vi "UI-SelfCheck.vi"() -> ()   [LabVIEW 2014]
panel:
  in  "error in (no error)":errorcluster caption="错误输入（无错误）"
  out "error out":errorcluster caption="错误输出"
  out "数据采集系统":string
  out "拖动系统":string
  out "齿轮系统":string
  out "液压系统":string
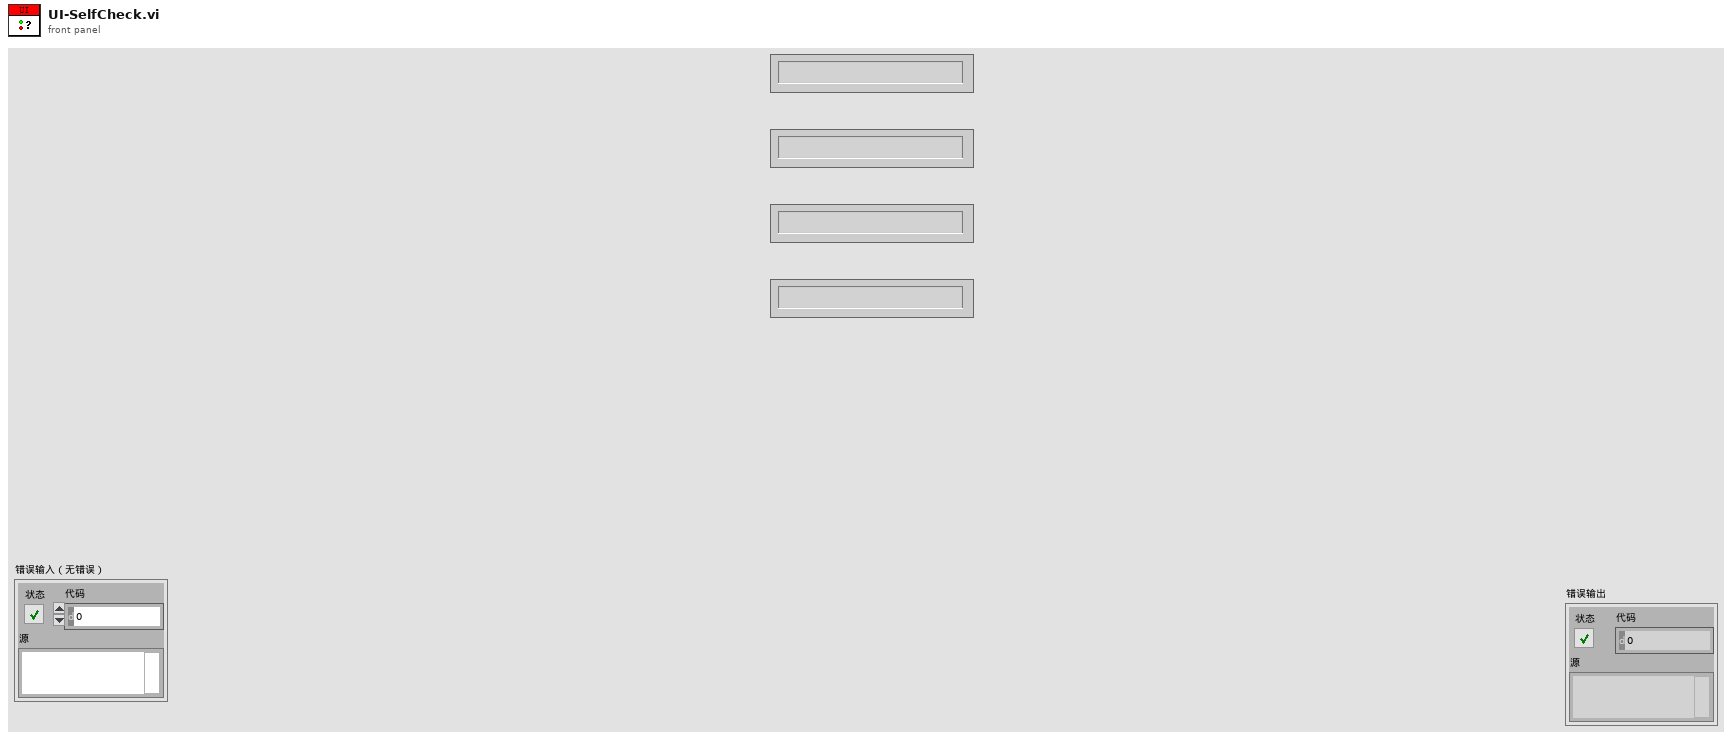
[diagram p1: front panel]
types:
  T1 = enum32{"Invalid", "Standard", "Closed", "Hidden", "Minimized", "Maximized"}
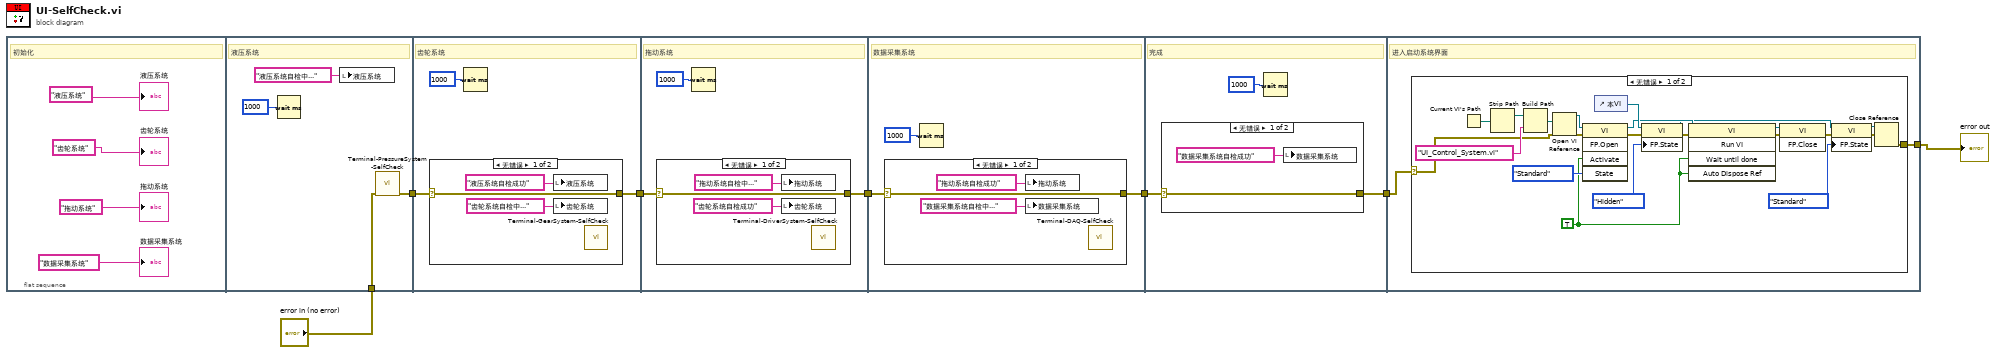
[diagram p0: block diagram]
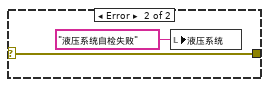
[diagram p2: hidden frame]
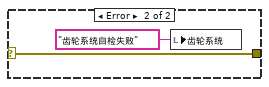
[diagram p3: hidden frame]
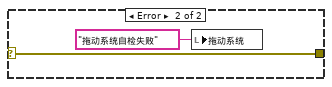
[diagram p4: hidden frame]
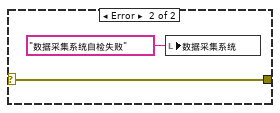
[diagram p5: hidden frame]
diagram:
  n1 = flat-sequence {
    tunnel: [w15] -> w7
    tunnel: "error in (no error)" -> [w12]
    tunnel: w7 -> [w18]
    tunnel: [w16] -> w6
    tunnel: w6 -> [w25]
    tunnel: [w24] -> w5
    tunnel: w5 -> [w33]
    tunnel: [w32] -> w3
    tunnel: w3 -> [w42]
    tunnel: [w41] -> w2
    tunnel: w2 -> [w48]
    tunnel: [w47] -> w1
    frame #0 {
      # "初始化"
      "数据采集系统" <- "数据采集系统"
      "拖动系统" <- "拖动系统"
      "齿轮系统" <- "齿轮系统"
      "液压系统" <- "液压系统"
    }
    frame #1 {
      # "液压系统"
      n2 = Wait (ms)(milliseconds to wait=u32 1000 ("等待时间（毫秒）")) -> ()  [unwired: 1 out]
      n3 = local write "液压系统"("液压系统自检中...") -> ()
      n4 = call "Terminal-PressureSystem-SelfCheck.vi"("error in (no error)"=w12) -> ("error out"=w15:errorcluster)  [unwired: 10 in]
    }
    frame #2 {
      # "齿轮系统"
      n5 = case shown="无错误" w18 {
        selector: w18 -> [w19 w22]
        tunnel: [w19 w22] -> w16
        frame No Error {
          n6 = local write "液压系统"("液压系统自检成功") -> ()
          n7 = local write "齿轮系统"("齿轮系统自检中...") -> ()
          n8 = call "Terminal-GearSystem-SelfCheck.vi"() -> ()  [unwired: 11 in, 1 out]
        }
        frame Error {
          n9 = local write "液压系统"("液压系统自检失败") -> ()
        }
      }
      n10 = Wait (ms)(milliseconds to wait=u32 1000 ("等待时间（毫秒）")) -> ()  [unwired: 1 out]
    }
    frame #3 {
      # "拖动系统"
      n11 = case shown="无错误" w25 {
        selector: w25 -> [w27 w30]
        tunnel: [w27 w30] -> w24
        frame No Error {
          n12 = local write "拖动系统"("拖动系统自检中...") -> ()
          n13 = local write "齿轮系统"("齿轮系统自检成功") -> ()
          n14 = call "Terminal-DriverSystem-SelfCheck.vi"() -> ()  [unwired: 11 in, 1 out]
        }
        frame Error {
          n15 = local write "齿轮系统"("齿轮系统自检失败") -> ()
        }
      }
      n16 = Wait (ms)(milliseconds to wait=u32 1000 ("等待时间（毫秒）")) -> ()  [unwired: 1 out]
    }
    frame #4 {
      # "数据采集系统"
      n17 = case shown="无错误" w33 {
        selector: w33 -> [w35 w38]
        tunnel: [w35 w38] -> w32
        frame No Error {
          n18 = local write "拖动系统"("拖动系统自检成功") -> ()
          n19 = local write "数据采集系统"("数据采集系统自检中...") -> ()
          n20 = call "Terminal-DAQ-SelfCheck.vi"() -> ()  [unwired: 11 in, 1 out]
        }
        frame Error {
          n21 = local write "拖动系统"("拖动系统自检失败") -> ()
        }
      }
      n22 = Wait (ms)(milliseconds to wait=u32 1000 ("等待时间（毫秒）")) -> ()  [unwired: 1 out]
    }
    frame #5 {
      # "完成"
      n23 = case shown="无错误" w42 {
        selector: w42 -> [w44 w46]
        tunnel: [w44 w46] -> w41
        frame No Error {
          n24 = local write "数据采集系统"("数据采集系统自检成功") -> ()
        }
        frame Error {
          n25 = local write "数据采集系统"("数据采集系统自检失败") -> ()
        }
      }
      n26 = Wait (ms)(milliseconds to wait=u32 1000 ("等待时间（毫秒）")) -> ()  [unwired: 1 out]
    }
    frame #6 {
      # "进入启动系统界面"
      n27 = case shown="无错误" w48 {
        selector: w48 -> [w50 w71]
        tunnel: [w49 w71] -> w47
        frame No Error {
          w53 = TRUE ("激活？")
          n28 = Current VI's Path() -> (path=w69:path)
          n29 = Strip Path(path=w69) -> (stripped path=w68:path)  [unwired: 1 out]
          n30 = Build Path(base path=w68, name or relative path="UI_Control_System.vi" ("名称或相对路径")) -> (appended path=w70:path)
          n31 = Open VI Reference(vi path=w70, error in (no error)=w50) -> (vi reference=w66:refnum<vi>, error out=w65:errorcluster)  [unwired: 4 in]
          n32 = invoke class="VI" method="FP.Open"(reference=w66, error in=w65, "Activate"=w53, "State"=T1."Standard" ("状态")) -> (reference out=w57:refnum<vi>, error out=w60:errorcluster)  [unwired: 1 in, 3 out]
          n33 = control-ref of="本VI"() -> (w61:refnum<vi>)
          n34 = property class="VI"(reference=w61, error in=w60, "FP.State"=T1."Hidden" ("前面板窗口:状态")) -> (reference out=w56:refnum<vi>, error out=w58:errorcluster)
          n35 = invoke class="VI" method="Run VI"(reference=w57, error in=w58, "Wait until done"=w53, "Auto Dispose Ref"=w53) -> (reference out=w63:refnum<vi>, error out=w62:errorcluster)  [unwired: 1 in, 3 out]
          n36 = invoke class="VI" method="FP.Close"(reference=w63, error in=w62) -> (error out=w55:errorcluster)  [unwired: 1 in, 2 out]
          n37 = property class="VI"(reference=w56, error in=w55, "FP.State"=T1."Standard" ("前面板窗口:状态")) -> (reference out=w52:refnum<vi>, error out=w51:errorcluster)
          n38 = Close Reference(reference=w52, error in (no error)=w51) -> (error out=w49:errorcluster)
        }
        frame Error {
        }
      }
    }
  }
  "error out" <- w1
